vi "Open Log11 emibin file.vi"(0 "file path":path, 11 "error in":errorcluster, 12 "File sub type(All)":u16=65535, 13 "Version(All)":u8=255) -> (2 "u8 std Array":T1[](array[typedef]), 3 "dbl Array":T2[](array[typedef]), 4 "refnum out":refnum<file>, 6 "Numb packages":i64, 8 "Log11 File Metrix":T3, 10 "Corrupt":bool, 15 "error out":errorcluster)   [LabVIEW 2011]
uses:
  Log11 emibin file Metrix.ctl
  Ch Info dbl.ctl
  Ch Info u8 std.ctl
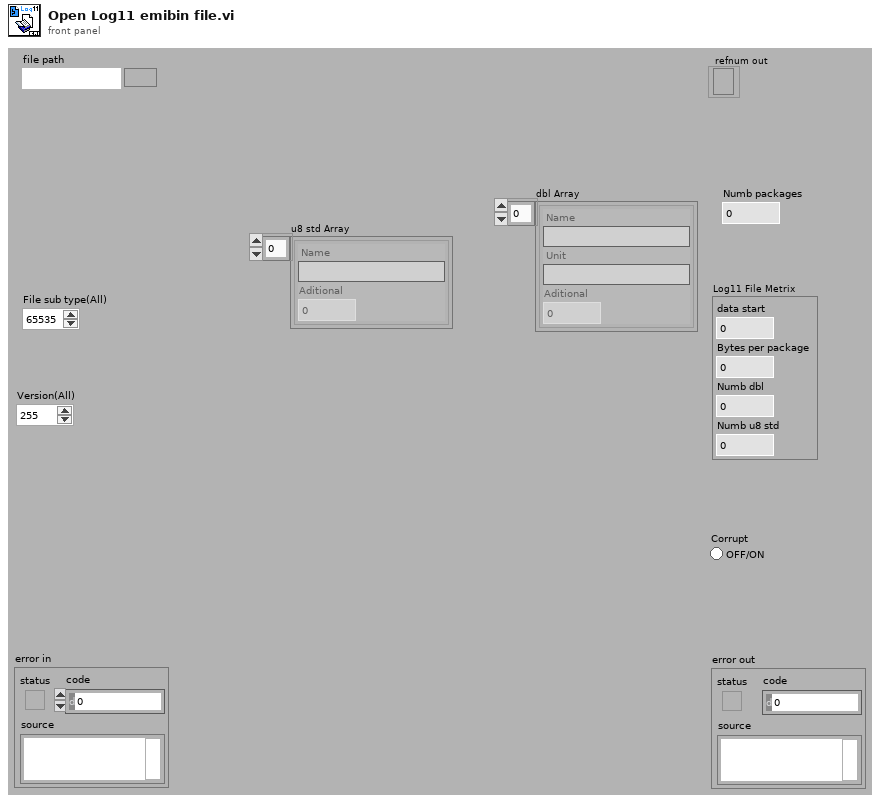
[diagram p1: front panel]
types:
  T1 = typedef "Ch Info u8 std.ctl" = cluster{"Name":string, "Aditional":i32}
  T2 = typedef "Ch Info dbl.ctl" = cluster{"Name":string, "Unit":string, "Aditional":i32}
  T3 = typedef "Log11 emibin file Metrix.ctl" = cluster{"data start":u32, "Bytes per package":i32, "Numb dbl":i32, "Numb u8 std":i32}
  T4 = enum16{"big-endian, network order", "native, host order", "little-endian"}
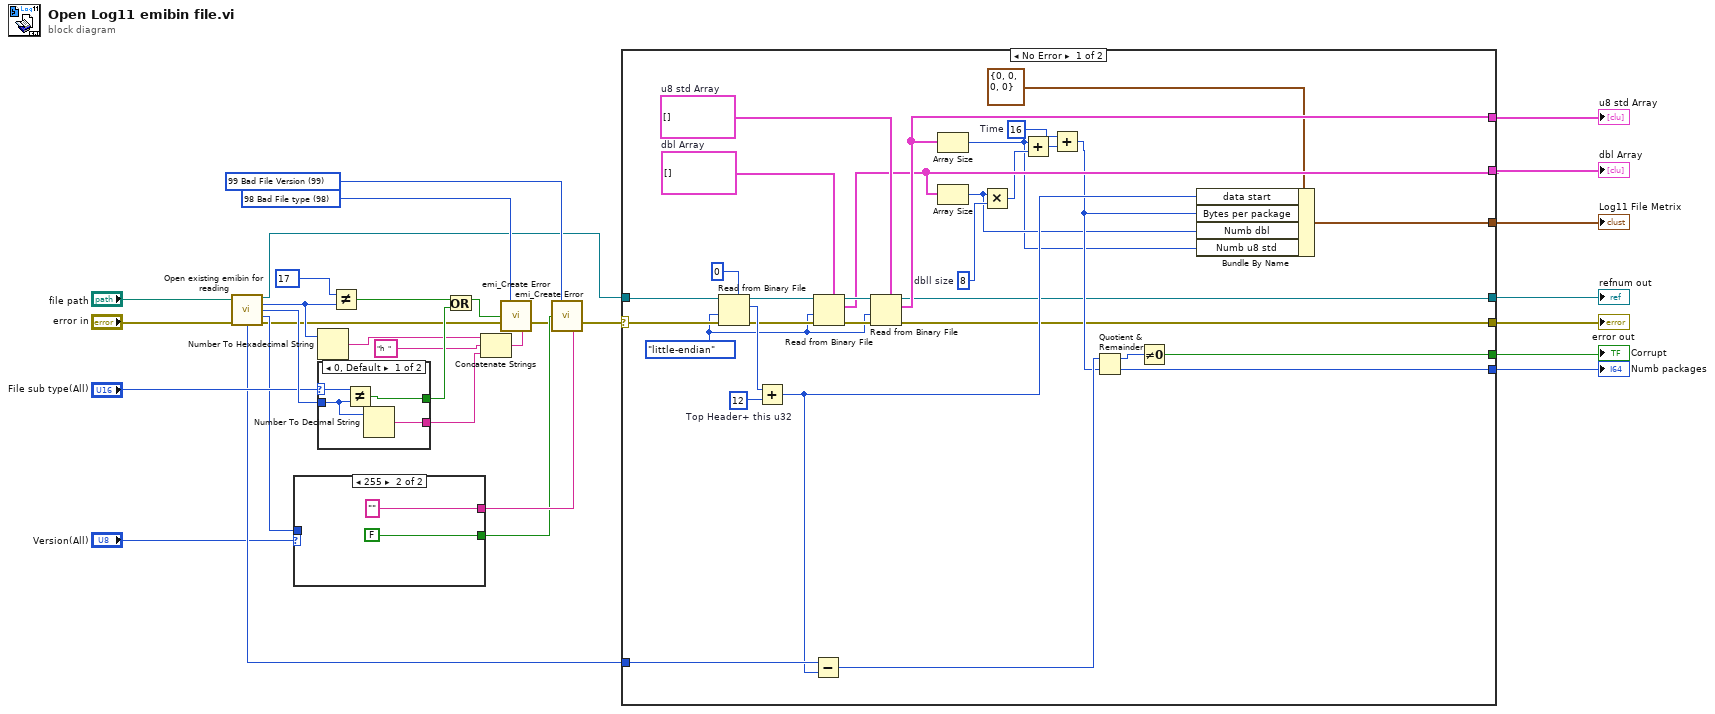
[diagram p0: block diagram]
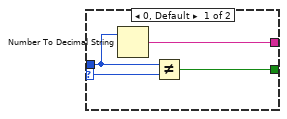
[diagram p2: hidden frame]
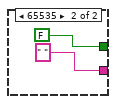
[diagram p3: hidden frame]
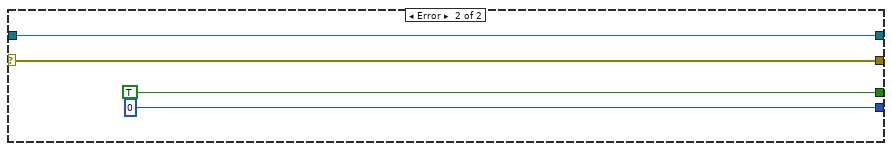
[diagram p4: hidden frame]
diagram:
  w17 = 99 items=["0 No Error"=0, "1 Invalid input parameter"=1, "6 Generic file IO "=6, "7 File not Found"=7, "35 Generic Pring Error"=35, "37 Device not Found"=37, "39 Device Unit Error"=39, "40 Could fot Open Device"=40, "42 Generic Error"=42, "52 Unknown Message"=52, "98 Bad File type"=98, "99 Bad File Version"=99, "100 Bad Data in File"=100, "1018 Unspecefied Error"=1018, "1041 Incorrect Password"=1041, "1043 Feature not in this version"=1043, "1109 Unsuported Data type"=1109, "1444 Did not close sucessfully"=1444] ("Error Code")
  w15 = 98 items=["0 No Error"=0, "1 Invalid input parameter"=1, "6 Generic file IO "=6, "7 File not Found"=7, "35 Generic Pring Error"=35, "37 Device not Found"=37, "39 Device Unit Error"=39, "40 Could fot Open Device"=40, "42 Generic Error"=42, "52 Unknown Message"=52, "98 Bad File type"=98, "99 Bad File Version"=99, "100 Bad Data in File"=100, "1018 Unspecefied Error"=1018, "1041 Incorrect Password"=1041, "1043 Feature not in this version"=1043, "1109 Unsuported Data type"=1109, "1444 Did not close sucessfully"=1444] ("Error Code")
  n1 = call "Open existing emibin for reading.vi"("file path"="file path", "error in (no error)"="error in") -> ("refnum out"=w12:refnum<file>, "File type Std"=w20:u8, "File type ID"=w30:u16, "File type Version"=w24:u8, "size (in bytes)"=w4:i64, "error out"=w13:errorcluster)  [unwired: 6 in, 2 out]
  n2 = case shown="255" "Version(All)" {
    selector: "Version(All)" -> [w32 _]
    tunnel: [w35 ""] -> w25
    tunnel: w24 -> [w34 _]
    tunnel: [w33 FALSE] -> w19
    frame 0, Default {
      n3 = Number To Decimal String(number=w34) -> (decimal integer string=w35:string)  [unwired: 1 in]
      n4 = Not Equal?(x=w34, y=w32) -> (x != y?=w33:bool)
    }
    frame 255 {
    }
  }
  n5 = Number To Hexadecimal String(2:w20) -> (0:w21:string)  [unwired: 1 in]
  n6 = case shown="0, Default" "File sub type(All)" {
    selector: "File sub type(All)" -> [w41 _]
    tunnel: [w38 " " ("string")] -> w27
    tunnel: [w40 FALSE] -> w29
    tunnel: w30 -> [w39 _]
    frame 0, Default {
      n7 = Not Equal?(x=w41, y=w39) -> (x != y?=w40:bool)
      n8 = Number To Decimal String(number=w39) -> (decimal integer string=w38:string)  [unwired: 1 in]
    }
    frame 65535 {
    }
  }
  n9 = Not Equal?(x=u8 17, y=w20) -> (x != y?=w18:bool)
  n10 = Or(x=w18, y=w29) -> (x .or. y?=w28:bool)
  n11 = Concatenate Strings(w21, "h  " ("string"), w27) -> (w23:string)
  n12 = call "emi_Create Error.vi"("Error Code"=w15, "Error(T)"=w28, "error in (no error)"=w13, "Append String(\"\")"=w23) -> ("error out"=w16:errorcluster)  [unwired: 11 in]
  n13 = call "emi_Create Error.vi"("Error Code"=w17, "Error(T)"=w19, "error in (no error)"=w16, "Append String(\"\")"=w25) -> ("error out"=w31:errorcluster)  [unwired: 11 in]
  n14 = case shown="No Error" w31 {
    selector: w31 -> [w74 w78]
    tunnel: [w46 w78] -> w2
    tunnel: [w45 w77] -> w3
    tunnel: w12 -> [w73 w77]
    tunnel: w4 -> [w55 _]
    tunnel: [w63 _] -> w8
    tunnel: [w62 _] -> w9
    tunnel: [w53 i64 0] -> w5
    tunnel: [w56 TRUE] -> w7
    tunnel: [w44 _] -> w11
    frame No Error {
      w58 = 16  # Time
      w61 = 8  # dbll size
      w52 = T4."little-endian" ("byte order (0:big-endian, network order)")
      w64 = T1[] []  # u8 std Array
      w67 = T2[] []  # dbl Array
      w70 = u32 12  # Top Header+ this u32
      n15 = Read from Binary File(5:u32 0 ("unsigned 32bit integer"), 8:w74, 9:w52, 11:w73) -> (0:w69:errorcluster, 2:w71:u32, 3:w68:refnum<file>)  [unwired: 2 in, 1 out]
      n16 = Add(x=w71, y=w70) -> (x+y=w50:u32)
      n17 = Subtract(x=w55, y=w50) -> (x-y=w60:i64)
      n18 = Read from Binary File(5:w67, 8:w69, 9:w52, 11:w68) -> (0:w66:errorcluster, 2:w62:T2[], 3:w65:refnum<file>)  [unwired: 2 in, 1 out]
      n19 = Read from Binary File(5:w64, 8:w66, 9:w52, 11:w65) -> (0:w46:errorcluster, 2:w63:T1[], 3:w45:refnum<file>)  [unwired: 2 in, 1 out]
      n20 = Array Size(array=w63) -> (size(s)=w47:i32)
      n21 = Array Size(array=w62) -> (size(s)=w48:i32)
      n22 = Multiply(x=w48, y=w61) -> (x*y=w54:i32)
      n23 = Add(x=w47, y=w54) -> (x+y=w59:i32)
      n24 = Add(x=w58, y=w59) -> (x+y=w49:i32)
      n25 = Quotient & Remainder(x=w60, y=w49) -> (x-y*floor(x/y)=w57:i64, floor(x/y)=w53:i64)
      n26 = Not Equal To 0?(x=w57) -> (x != 0?=w56:bool)
      n27 = Bundle By Name(cluster=T3 {"data start"=0, "Bytes per package"=0, "Numb dbl"=0, "Numb u8 std"=0} ("Log11 File Metrix"), "data start"=w50, "Bytes per package"=w49, "Numb dbl"=w48, "Numb u8 std"=w47) -> (w44:T3)
    }
    frame Error {
    }
  }
  "Log11 File Metrix" <- w11
  "dbl Array" <- w9
  "u8 std Array" <- w8
  "Corrupt" <- w7
  "Numb packages" <- w5
  "refnum out" <- w3
  "error out" <- w2
